vi "Write name.vi"(8 "error in (no error)":errorcluster, 10 "name":string, 11 "GSdevice in":refnum<class "GSdevice.lvclass">) -> (0 "error out":errorcluster, 3 "GSdevice out":refnum<class "GSdevice.lvclass">)   [LabVIEW 2018, in "GSdevice.lvclass"]
uses:
  GSdevice.lvclass
  GSdevice.lvclass/GSdevice.ctl
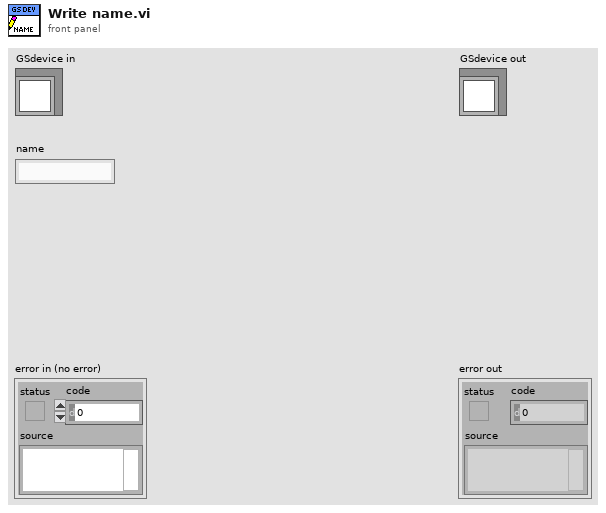
[diagram p1: front panel]
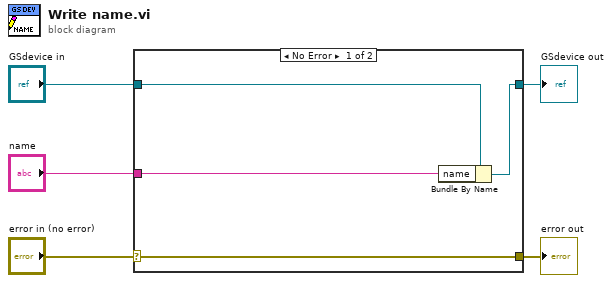
[diagram p0: block diagram]
diagram:
  n1 = case shown="No Error" "error in (no error)" {
    selector: "error in (no error)" -> [w9 w10]
    tunnel: [w9 w10] -> w4
    tunnel: [w7 w11] -> w2
    tunnel: "GSdevice in" -> [w8 w11]
    tunnel: "name" -> [w6 _]
    frame No Error {
      n2 = Bundle By Name(cluster=w8, "name"=w6) -> (w7:refnum<class "GSdevice.lvclass">)
    }
    frame Error {
    }
  }
  "error out" <- w4
  "GSdevice out" <- w2
